vi "NI-Digital Loopback and Compare.vi"() -> ()   [LabVIEW 2021]
doc: "Overview\nDemonstrates how to use the NI-Digital Pattern Driver API to create and configure an instrument session and to burst a pattern on the digital pattern instrument, while checking for pass/fail conditions in a loopback configuration."
uses:
  <instrlib>/niDigital/niDigital.llb/niDigital Burst Pattern (Pass Fail).vi
  <instrlib>/niDigital/niDigital.llb/niDigital Selected Function.ctl
  <instrlib>/niDigital/niDigital.llb/niDigital Load Specifications Levels and Timing (Single).vi
panel:
  in  "Simulate?":bool=TRUE
  in  "resource name":refnum<k15>="PXI1Slot2,PXI1Slot3"
  out "pass":bool[](array[boolean])
  # "Overview\nDemonstrates how to use the NI-Digital Pattern Driver API to create and configure an instrument session and to burst a pattern on the digital pattern instrument, while checking for pass/fail conditions in a loopback configuration.\n\nInstructions\n1. Connect the digital pattern instrument(s) in loopback configuration.\n    - Connect physical channel 0 to channel 6.\n    - Connect physical channel 1 to channel 7.\n2. Use the resource name control to select the digital pattern instrument. Ensure that the instrument name in the PinMap.pinmap file matches the resource name of the digital pattern instrument. The default value for the resource name is \"PXI1Slot2,PXI1Slot3\".\n3. Run the VI. The pass indicator displays results.\n4. To run on hardware deselect Simulate?  and modify the resource name as appropriate."
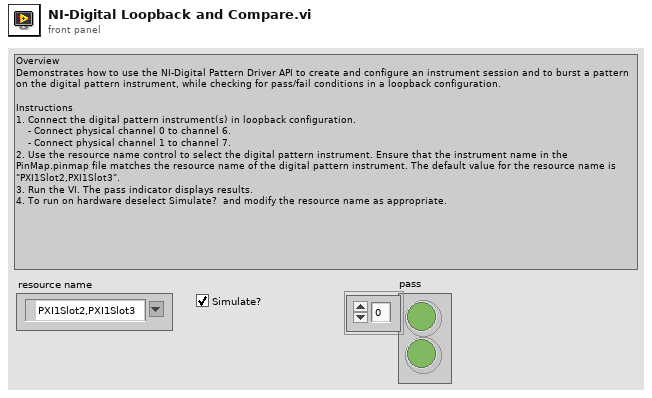
[diagram p1: front panel]
types:
  T1 = typedef "niDigital Selected Function.ctl" = i32
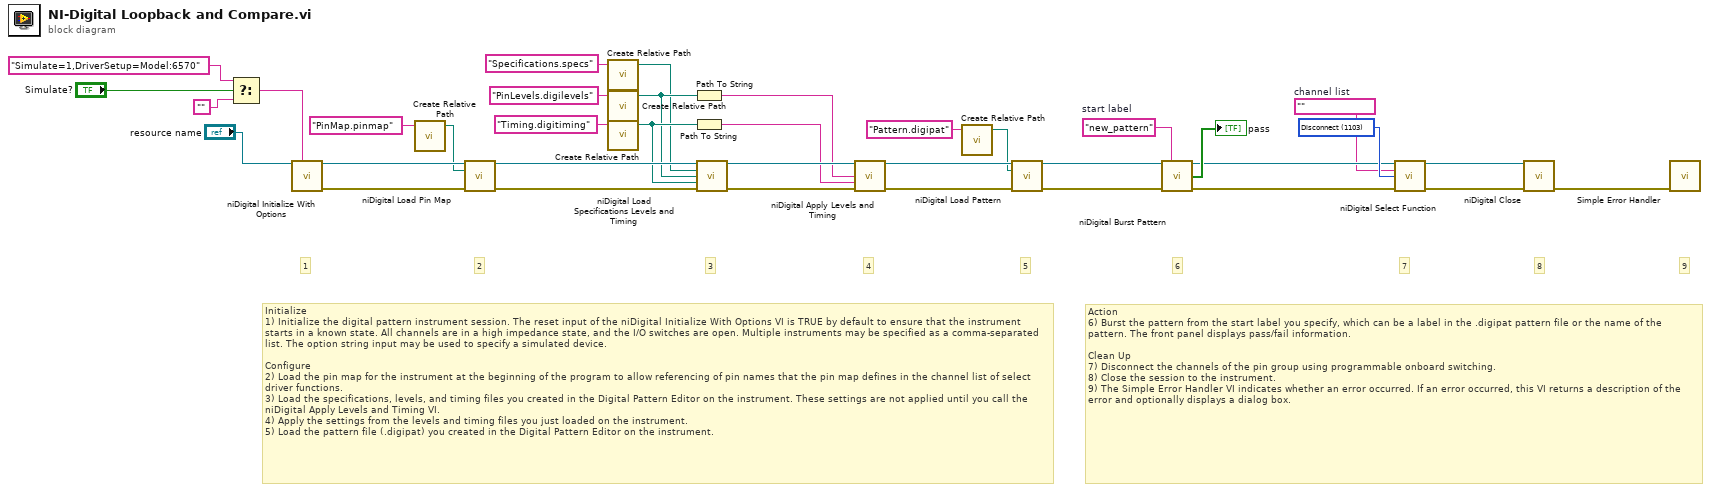
[diagram p0: block diagram]
diagram:
  w25 = T1 1103 items=["Digital"=1100, "PPMU"=1101, "Off"=1102, "Disconnect"=1103] ("function")
  w20 = ""  # channel list
  w31 = "new_pattern"  # start label
  # "7"
  # "Action\n6) Burst the pattern from the start label you specify, which can be a label in the .digipat pattern file or the name of the pattern. The front panel displays pass/fail information.\n \nClean Up\n7) Disconnect the channels of the pin group using programmable onboard switching. \n8) Close the session to the instrument.\n9) The Simple Error Handler VI indicates whether an error occurred. If an error occurred, this VI returns a description of the error and optionally displays a dialog box."
  # "Initialize\n1) Initialize the digital pattern instrument session. The reset input of the niDigital Initialize With Options VI is TRUE by default to ensure that the instrument starts in a known state. All channels are in a high impedance state, and the I/O switches are open. Multiple instruments may be specified as a comma-separated list. The option string input may be used to specify a simulated device.\n\nConfigure\n2) Load the pin map for the instrument at the beginning of the program to allow referencing of pin names that the pin map defines in the channel list of select driver functions.\n3) Load the specifications, levels, and timing files you created in the Digital Pattern Editor on the instrument. These settings are not applied until you call the niDigital Apply Levels and Timing VI.\n4) Apply the settings from the levels and timing files you just loaded on the instrument.\n5) Load the pattern file (.digipat) you created in the Digital Pattern Editor on the instrument."
  # "9"
  # "8"
  # "6"
  # "5"
  # "4"
  # "3"
  # "2"
  # "1"
  n1 = Select(t="Simulate=1,DriverSetup=Model:6570", s="Simulate?", f="") -> (s? t:f=w2:string)
  n2 = call <instrlib>:"niDigital Initialize With Options.vi"("resource name"="resource name", "option string"=w2) -> ("instrument handle"=w30:refnum<k15>, "error out"=w29:errorcluster)  [unwired: 12 in]
  n3 = call "Create Relative Path.vi"("file name"="PinMap.pinmap" ("name or relative path")) -> ("appended path"=w12:path)  [unwired: 4 in]
  n4 = call <instrlib>:"niDigital Load Pin Map.vi"("instrument handle"=w30, "pin map file"=w12, "error in"=w29) -> ("instrument handle out"=w28:refnum<k15>, "error out"=w27:errorcluster)  [unwired: 11 in]
  n5 = call "Create Relative Path.vi"("file name"="Specifications.specs" ("name or relative path")) -> ("appended path"=w6:path)  [unwired: 4 in]
  n6 = call "Create Relative Path.vi"("file name"="PinLevels.digilevels" ("name or relative path")) -> ("appended path"=w10:path)  [unwired: 4 in]
  n7 = call "Create Relative Path.vi"("file name"="Timing.digitiming" ("name or relative path")) -> ("appended path"=w11:path)  [unwired: 4 in]
  n8 = Path To String(path=w10) -> (string=w9:string)
  n9 = Path To String(path=w11) -> (string=w8:string)
  n10 = call-poly <instrlib>:"niDigital Load Specifications Levels and Timing.vi"("instrument handle"=w28, "specifications file path"=w6, "levels file path"=w10, "timing file path"=w11, "error in"=w27) -> ("instrument handle out"=w36:refnum<k15>, "error out"=w35:errorcluster)  [unwired: 9 in]
  n11 = call <instrlib>:"niDigital Apply Levels and Timing.vi"("instrument handle"=w36, "levels sheet"=w9, "timing sheet"=w8, "error in"=w35) -> ("instrument handle out"=w33:refnum<k15>, "error out"=w34:errorcluster)  [unwired: 10 in]
  n12 = call "Create Relative Path.vi"("file name"="Pattern.digipat" ("name or relative path")) -> ("appended path"=w7:path)  [unwired: 4 in]
  n13 = call <instrlib>:"niDigital Load Pattern.vi"("instrument handle"=w33, "pattern file"=w7, "error in"=w34) -> ("instrument handle out"=w19:refnum<k15>, "error out"=w18:errorcluster)  [unwired: 11 in]
  n14 = call-poly <instrlib>:"niDigital Burst Pattern.vi"("instrument handle"=w19, "start label"=w31, "error in"=w18) -> ("instrument handle out"=w24:refnum<k15>, "pass"=→"pass":bool[], "error out"=w23:errorcluster)  [unwired: 10 in]
  n15 = call <instrlib>:"niDigital Select Function.vi"("instrument handle"=w24, "channel list"=w20, "function"=w25, "error in"=w23) -> ("instrument handle out"=w22:refnum<k15>, "error out"=w21:errorcluster)  [unwired: 10 in]
  n16 = call <instrlib>:"niDigital Close.vi"("instrument handle"=w22, "error in"=w21) -> ("error out"=w32:errorcluster)  [unwired: 13 in]
  n17 = call <vilib>:"Simple Error Handler.vi"("error in (no error)"=w32) -> ()  [unwired: 4 in, 5 out]
